vi "Ic_grating_pattern.vi"(6 "Row:0 or column:1":u32, 7 "Slip_factor":i32, 8 "error in (no error)":errorcluster, 9 "gradation width":u32=1, 10 "gradation number":u32=2, 11 "2D array in (LCOS size buf)":u8[][](array[numeric])=array128x128[16384 elements]) -> (0 "error out":errorcluster, 3 "2D array out":u8[][](array[numeric]))   [LabVIEW 2016]
uses:
  SLM_Control_VI_source/Image_Control.dll
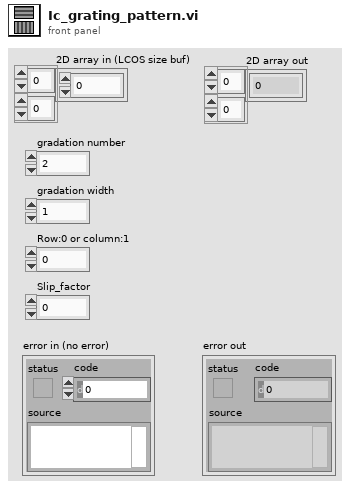
[diagram p1: front panel]
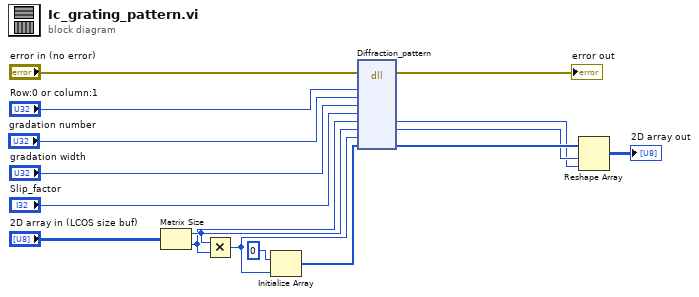
[diagram p0: block diagram]
diagram:
  n1 = Matrix Size(0:"2D array in (LCOS size buf)") -> (1:w12:i32, 2:w11:i32)
  n2 = Multiply(x=w12, y=w11) -> (x*y=w10:i32)
  n3 = Initialize Array(u8 0 ("要素"), w10) -> (w9:u8[])
  n4 = dll-call lib="C:/Users/hs5921/Desktop/SLM_Control_VI_source/Image_Control.dll" fn="Diffraction_pattern"(error in="error in (no error)", "Row0OrColumn1"="Row:0 or column:1", "gradationNumber"="gradation number", "gradationWidth"="gradation width", "Slip_factor"="Slip_factor", "X_pixel_target"=w11, "Y_pixel_target"=w12, "targetDataSize"=w10, "1DArrayOut"=w9) -> (error out=→"error out":errorcluster, "X_pixel_target"=w3:i32, "Y_pixel_target"=w4:i32, "1DArrayOut"=w5:u8[])  [unwired: 8 in, 1 out]
  n5 = Reshape Array(w5, w4, w3) -> (→"2D array out":u8[][])
